vi "Template-Actor-Library.vi"(8 "error in (no error)":errorcluster) -> (0 "error out":errorcluster, 3 "Template-Actor-Root":path)   [LabVIEW 2018, in "Scripting.lvlib"]
uses:
  Scripting.lvlib
  Tooling-Root.vi
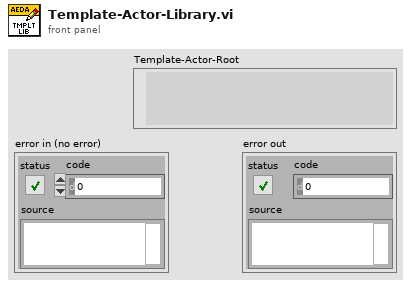
[diagram p1: front panel]
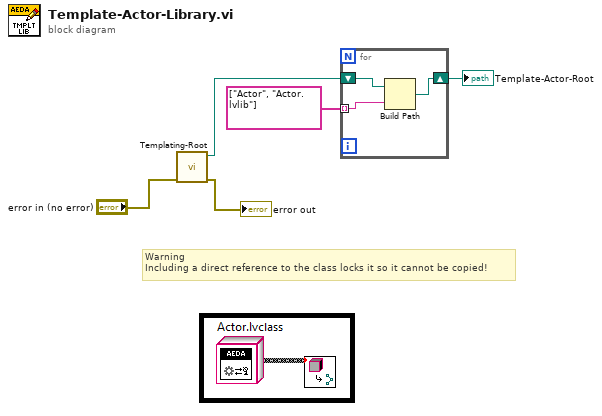
[diagram p0: block diagram]
diagram:
  # "Warning\nIncluding a direct reference to the class locks it so it cannot be copied!"
  n1 = call "Templating-Root.vi"("error in (no error)"="error in (no error)") -> ("error out"=→"error out":errorcluster, "Template-Root"=w2:path)  [unwired: 9 in]
  n2 = for {
    shift-right: [w8] -> w3
    shift-left: w2 -> [w7]
    tunnel: string[] ["Actor", "Actor.lvlib"] -> [w6] mode=indexing
    n3 = Build Path(base path=w7, name or relative path=w6) -> (appended path=w8:path)
  }
  "Template-Actor-Root" <- w3
